vi "Move along Curve.vi"(4 "Destination Angle":dbl=nan, 5 "direction":u16(ring) items=["Clockwise", "Counter-clockwise"], 6 "Radius":dbl=5.0, 8 "error in":errorcluster, 9 "Speed":dbl=5.0, 10 "Destination":refnum<class "Vec3d.lvclass">, 11 "Gantry in":refnum<class "Gantry.lvclass">) -> (0 "error out":errorcluster, 3 "Gantry out":refnum<class "Gantry.lvclass">)   [LabVIEW 2026, in "Gantry.lvclass"]
uses:
  Gantry.lvclass
  Vec3d Class/Vec3d.lvclass
  Gantry.lvclass/Gantry.ctl
  <instrlib>/Aerotech Automation1/Tasks/Task State.ctl
  <instrlib>/Aerotech Automation1/Aerotech Automation1.lvlib
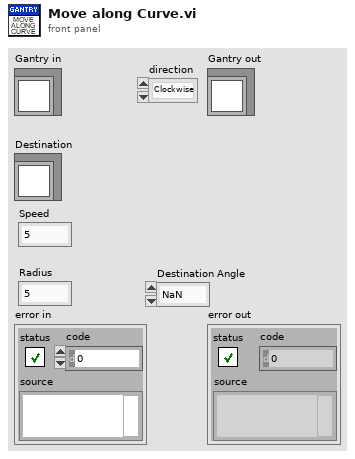
[diagram p1: front panel]
types:
  T1 = typedef "Aerotech Automation1.lvlib/Task State.ctl" = enum16{"Unavailable", "Inactive", "Idle", "ProgramReady", "ProgramRunning", "ProgramFeedhold", "ProgramPaused", "ProgramComplete", "Error", "Queue"}
  T2 = typedef "TaskStatus.ctl" = cluster{"Task Status0 (num)":i32, "Task Status0 (bits)":cluster{"CallbackHoldActive":bool, "CallbackResponding":bool, "CannedFunctionExecuting":bool, "CornerRounding":bool, "FeedHoldActive":bool, "ImmediateConcurrent":bool, "ImmediateExecuting":bool, "InterruptMotionActive":bool, "JoystickActive":bool, "JoystickLowSpeedActive":bool, "None":bool, "PendingAxesStop":bool, "ProbeCycle":bool, "ProgramAssociated":bool, "ProgramControlRestricted":bool, "ProgramReset":bool, "Retrace":bool, "ReturnMotionExecuting":bool, "SingleStepInto":bool, "SingleStepOver":bool, "SoftHomeActive":bool, "SoftwareESTOPActive":bool, "SpindleActive0":bool, "SpindleActive1":bool, "SpindleActive2":bool, "SpindleActive3":bool}, "Task Status0 (str)":string, "Task Status1 (num)":i32, "Task Status1 (bits)":cluster{"AsyncSMCMotionAbortPending":bool, "CannedFunctionPending":bool, "CutterOffsetsDisabling":bool, "CutterOffsetsEnablingNegative":bool, "CutterOffsetsEnablingPositive":bool, "CutterRadiusDisabling":bool, "CutterRadiusEnabling":bool, "FeedHeldAxesStopped":bool, "GalvoIFVDeactivationPending":bool, "IFOVBufferHold":bool, "Interrupted":bool, "MotionModeAbsOffsets":bool, "MSOChange":bool, "NoMFOFloor":bool, "None":bool, "OnGosubPending":bool, "ProgramStopPending":bool, "RetraceRequested":bool, "SpindleFeedHeld":bool}, "Task Status1 (str)":string, "Task Status2 (num)":i32, "Task Status2 (bits)":cluster{"Coord1Plane1":bool, "Coord1Plane2":bool, "Coord1Plane3":bool, "Coord2Plane1":bool, "Coord2Plane2":bool, "Coord2Plane3":bool, "CutterOffsetsActiveNeg":bool, "CutterOffsetsActivePos":bool, "CutterRadiusActiveLeft":bool, "CutterRadiusActiveRight":bool, "LimitFeedRateActive":bool, "LimitMFOActive":bool, "MirrorActive":bool, "MotionContinuousActive":bool, "MotionFiber":bool, "MotionModeCCW":bool, "MotionModeCoordinated":bool, "MotionModeCW":bool, "MotionModeRapid":bool, "MotionPVT":bool, "None":bool, "NormalcyActiveLeft":bool, "NormalcyActiveRight":bool, "NormalcyAlignment":bool, "OffsetFixtureActive":bool, "ProfileActive":bool, "RotationActive":bool, "RThetaCylindricalActive":bool, "RThetaPolarActive":bool, "ScalingActive":bool}, "Task Status2 (str)":string, "Task Mode (num)":i32, "Task Mode (bits)":cluster{"Absolute":bool, "AccelModeRate":bool, "AccelTypeLinear":bool, "AccelTypeScurve":bool, "AutoMode":bool, "BlockDelete":bool, "BlockDelete2":bool, "DecelModeRate":bool, "DecelTypeLinear":bool, "DecelTypeScurve":bool, "InverseCircular":bool, "InverseDominance":bool, "MFOActiveOnJog":bool, "MFOLock":bool, "Minutes":bool, "MotionContinuous":bool, "MSOLock":bool, "None":bool, "OptionalPause":bool, "OverMode":bool, "ProgramFeedRateMPU":bool, "ProgramFeedRateUPR":bool, "Secondary":bool, "SpindleStopOnProgramHalt":bool, "WaitAuto":bool, "WaitForInPos":bool}, "Task Mode (str)":string, "Queue Status (num)":i32, "Queue Status (bits)":cluster{"None":bool, "QueueBufferEmpty":bool, "QueueBufferFull":bool, "QueueBufferPaused":bool, "QueueBufferStarted":bool, "QueueLargeProgramExecuting":bool, "QueueModeActive":bool}, "Queue Status (str)":string, "Task State":i32}
  T3 = typedef "Aerotech Automation1.lvlib/Task Status Cluster.ctl" = cluster{"TaskState":T1, "TaskMode":i32, "AeroScriptSourceFileName":string, "CompiledAeroScriptFileName":string, "ManualFeedrateOverride":dbl, "Warning Number":i32, "Warning Message":string, "Error Number":i32, "Error Message":string}
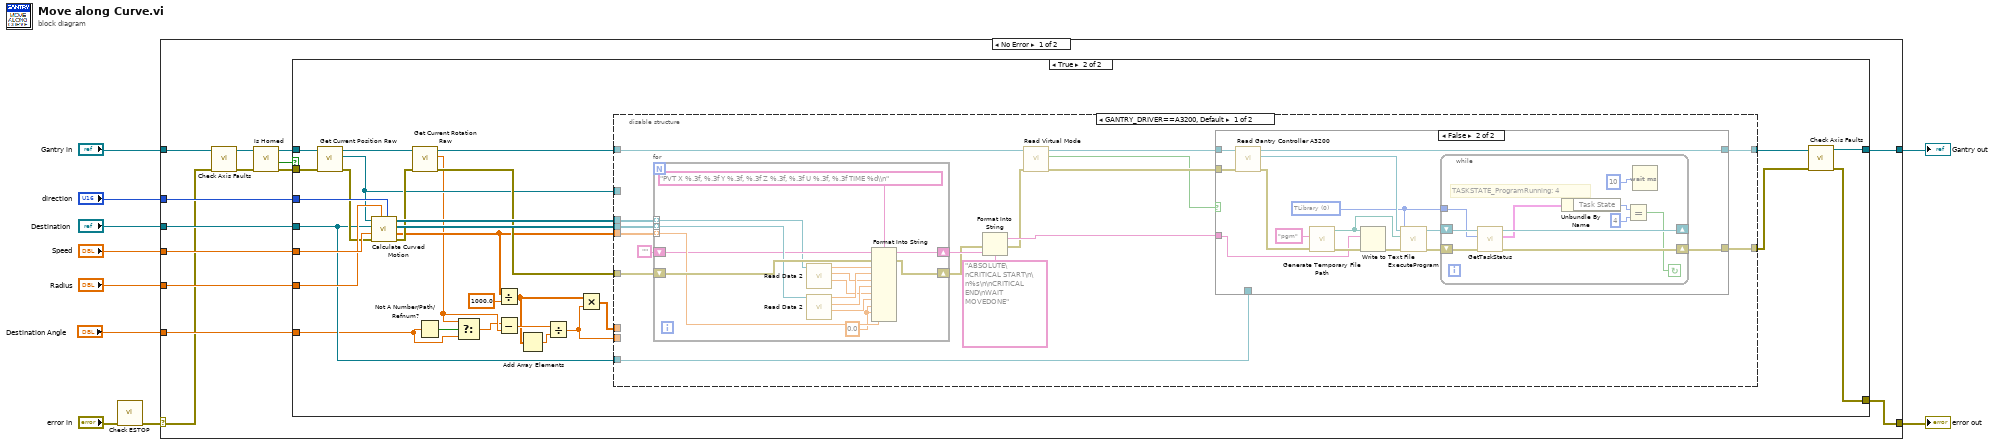
[diagram p0: block diagram]
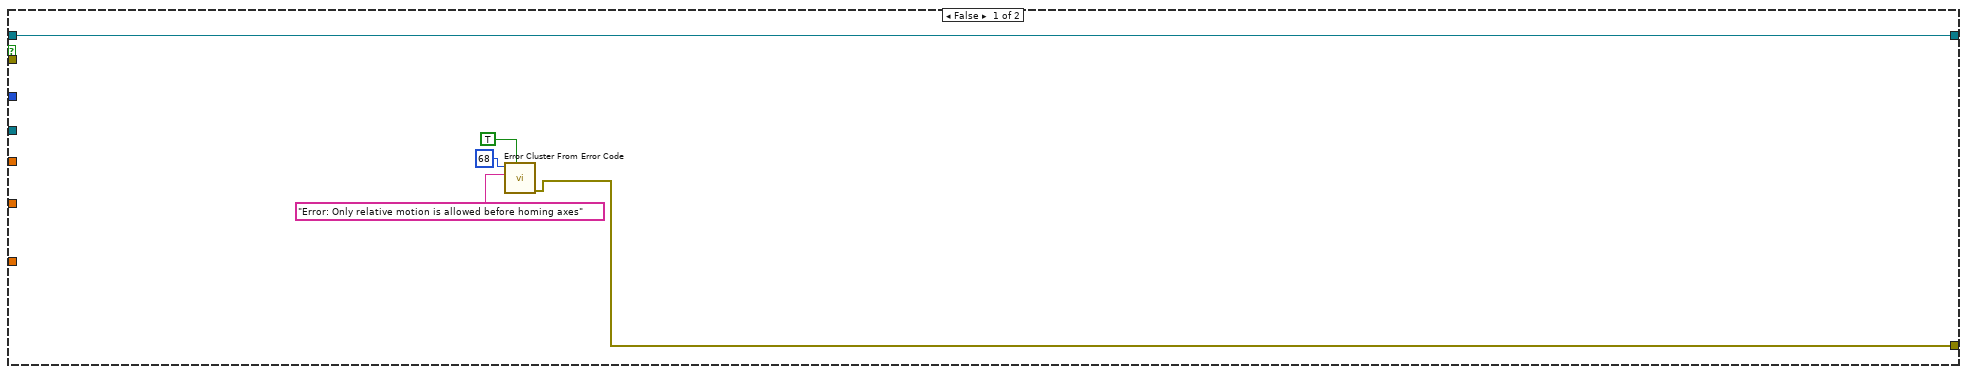
[diagram p2: hidden frame]
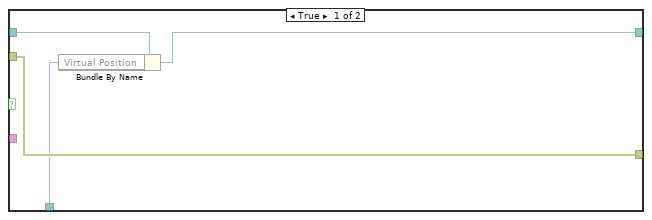
[diagram p3: hidden frame]
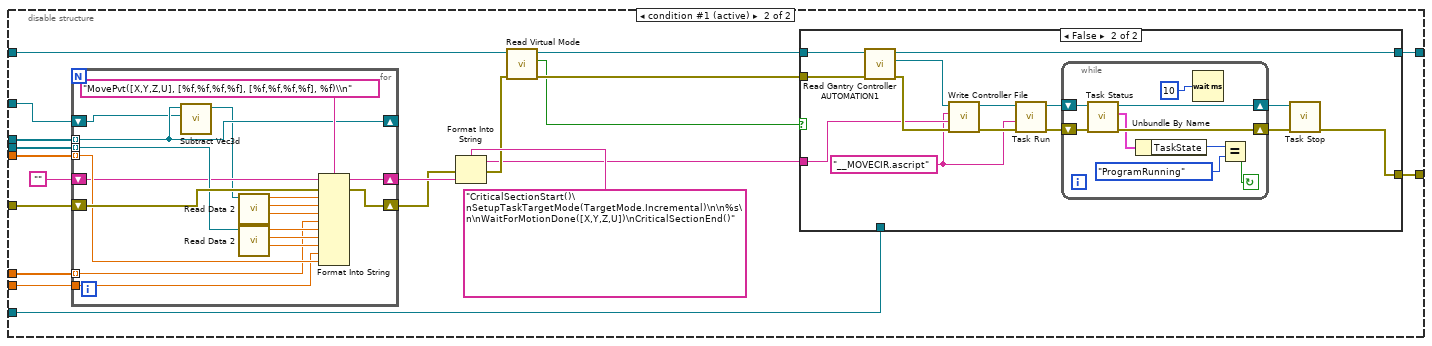
[diagram p4: hidden frame]
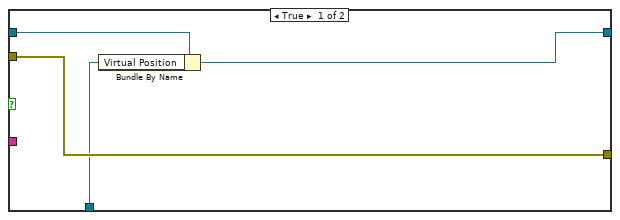
[diagram p5: hidden frame]
diagram:
  n1 = call "Check ESTOP.vi"("error in"="error in") -> ("error out"=w5:errorcluster)  [unwired: 10 in]
  n2 = case shown="No Error" w5 {
    selector: w5 -> [w14 w185]
    tunnel: [w21 w185] -> w10
    tunnel: [w22 w184] -> w9
    tunnel: "Gantry in" -> [w12 w184]
    tunnel: "Destination" -> [w24 _]
    tunnel: "Speed" -> [w23 _]
    tunnel: "direction" -> [w17 _]
    tunnel: "Radius" -> [w16 _]
    tunnel: "Destination Angle" -> [w15 _]
    frame No Error {
      n3 = call "Check Axis Faults.vi"("error in (no error)"=w14, "Gantry in"=w12) -> ("error out"=w13:errorcluster, "Gantry out"=w11:refnum<class "Gantry.lvclass">)  [unwired: 8 in]
      n4 = call "Is Homed.vi"("error in (no error)"=w13, "Gantry in"=w11) -> ("error out"=w18:errorcluster, "homed?"=w19:bool, "Gantry out"=w20:refnum<class "Gantry.lvclass">)  [unwired: 7 in]
      n5 = case shown="True" w19 {
        tunnel: w24 -> [_ w41]
        tunnel: w20 -> [w25 w43]
        tunnel: w23 -> [_ w58]
        tunnel: w18 -> [_ w42]
        tunnel: [w25 w54] -> w22
        tunnel: [w26 w52] -> w21
        tunnel: w17 -> [_ w56]
        tunnel: w16 -> [_ w57]
        tunnel: w15 -> [_ w32]
        frame False {
          n6 = call <vilib>:"Error Cluster From Error Code.vi"("show call chain? (False)"=TRUE, "error message (\"\")"="Error: Only relative motion is allowed before homing axes", "error code (0)"=68) -> ("error out"=w26:errorcluster)  [unwired: 6 in]
        }
        frame True {
          n7 = call-dynamic "Get Current Position Raw.vi"("error in"=w42, "Gantry in"=w43) -> ("error out"=w50:errorcluster, "Vec3d Class out"=w44:refnum<class "Vec3d.lvclass">, "Gantry out"=w51:refnum<class "Gantry.lvclass">)  [unwired: 7 in]
          n8 = call "Calculate Curved Motion.vi"("orientation"=w56, "Radius (mm)"=w57, "error in (no error)"=w50, "Speed (mm/s)"=w58, "Destination (mm)"=w41, "Origin (mm)"=w44) -> ("error out"=w46:errorcluster, "Times (ms)"=w36:dbl[], "Speeds (mm/s)"=w47:refnum<class "Vec3d.lvclass">[], "Coordinates (mm)"=w48:refnum<class "Vec3d.lvclass">[])  [unwired: 2 in]
          n9 = call-dynamic "Get Current Rotation Raw.vi"("error in"=w46, "Gantry in"=w51) -> ("error out"=w45:errorcluster, "Current Rotation"=w31:dbl, "Gantry out"=w49:refnum<class "Gantry.lvclass">)  [unwired: 7 in]
          n10 = Not A Number/Path/Refnum?(number/path/refnum=w32) -> (NaN/Path/Refnum?=w33:bool)
          n11 = Select(t=w31, s=w33, f=w32) -> (s? t:f=w30:dbl)
          n12 = Divide(x=w36, y=1000.0) -> (x/y=w34:dbl[])
          n13 = Subtract(x=w30, y=w31) -> (x-y=w40:dbl)
          n14 = Add Array Elements(numeric array=w34) -> (sum=w37:dbl)
          n15 = Divide(x=w40, y=w37) -> (x/y=w39:dbl)
          n16 = Multiply(x=w34, y=w39) -> (x*y=w38:dbl[])
          n17 = disable-structure shown="GANTRY_DRIVER==A3200, Default" {
            disable-tunnel: w49 -> [w66 w127]
            disable-tunnel: w48 -> [w65 w137]
            disable-tunnel: w47 -> [w64 w136]
            disable-tunnel: w36 -> [w63 w135]
            disable-tunnel: w45 -> [w62 w138]
            disable-tunnel: [w59 w131] -> w53
            disable-tunnel: [w60 w130] -> w55
            disable-tunnel: w44 -> [_ w129]
            disable-tunnel: w41 -> [w61 w122]
            disable-tunnel: w39 -> [_ w120]
            disable-tunnel: w38 -> [_ w119]
            frame condition #0 {
              n18 = for {
                shift-right: [w114] -> w71
                shift-left: w62 -> [w117]
                tunnel: w65 -> [w111] mode=indexing
                tunnel: w64 -> [w116] mode=indexing
                tunnel: w63 -> [w115] mode=indexing
                shift-right: [w112] -> w72
                shift-left: "" -> [w113]
                w104 = 0.0 ("input 4")
                n19 = call-dynamic "Read Data 2.vi"("Vec3d in"=w111) -> ("Z"=w106:dbl, "Y"=w108:dbl, "X"=w110:dbl)  [unwired: 7 in, 1 out]
                n20 = call-dynamic "Read Data 2.vi"("Vec3d in"=w116) -> ("Z"=w105:dbl, "Y"=w107:dbl, "X"=w109:dbl)  [unwired: 7 in, 1 out]
                n21 = Format Into String(format string="PVT X %.3f, %.3f Y %.3f, %.3f Z %.3f, %.3f U %.3f, %.3f TIME %d\\n", initial string=w113, error in=w117, w110, w109, w108, w107, w106, w105, w104, w104, w115) -> (resulting string=w112:string, error out=w114:errorcluster)
              }
              n22 = Format Into String(format string="ABSOLUTE\nCRITICAL START\n\n%s\n\nCRITICAL END\nWAIT MOVEDONE", error in=w71, w72) -> (resulting string=w74:string, error out=w69:errorcluster)  [unwired: 1 in]
              n23 = call-dynamic "Read Virtual Mode.vi"("error in (no error)"=w69, "Gantry in"=w66) -> ("error out"=w68:errorcluster, "Is Virtual"=w67:bool, "Gantry out"=w70:refnum<class "Gantry.lvclass">)  [unwired: 6 in, 1 out]
              n24 = case shown="False" w67 {
                tunnel: w74 -> [_ w87]
                tunnel: [w79 w81] -> w59
                tunnel: [w76 w93] -> w60
                tunnel: w70 -> [w78 w92]
                tunnel: w68 -> [w79 w91]
                tunnel: w61 -> [w77 _]
                frame True {
                  n25 = Bundle By Name(cluster=w78, "Virtual Position"=w77) -> (w76:refnum<class "Gantry.lvclass">)
                }
                frame False {
                  w80 = 0 items=["TLibrary", "T01", "T02", "T03", "T04", "T05", "T06", "T07", "T08", "T09", "T10", "T11", "T12", "T13", "T14", "T15", "T16", "T17", "T18", "T19", "T20", "T21", "T22", "T23", "T24", "T25", "T26", "T27", "T28", "T29", "T30", "T31"] ("taskId")
                  n26 = call "Read Gantry Controller A3200.vi"("error in (no error)"=w91, "Gantry in"=w92) -> ("error out"=w90:errorcluster, "A3200 controller out"=w86:refnum<k24>, "Gantry out"=w93:refnum<class "Gantry.lvclass">)  [unwired: 7 in]
                  n27 = call <vilib>:"Generate Temporary File Path.vi"("error in (no error)"=w90, "Temporary File Extension (tmp)"="pgm") -> ("error out"=w88:errorcluster, "Unique Temporary File Path"=w84:path)  [unwired: 8 in]
                  n28 = Write to Text File(file (use dialog)=w84, text=w87, error in=w88) -> (error out=w85:errorcluster)  [unwired: 1 in, 2 out]
                  n29 = call "ExecuteProgram.vi"("error in (no error)"=w85, "taskId"=w80, "program name and path"=w84, "controller in"=w86) -> ("error out"=w83:errorcluster, "controller out"=w82:refnum<k24>)  [unwired: 5 in, 1 out]
                  n30 = while {
                    shift-right: [w100] -> w81
                    shift-left: w83 -> [w102]
                    shift-right: [w101] -> _
                    shift-left: w82 -> [w103]
                    tunnel: w80 -> [w94]
                    stop <- w96 continue-if-true
                    # "TASKSTATE_ProgramRunning: 4"
                    n31 = call "GetTaskStatus.vi"("error in (no error)"=w102, "task"=w94, "controller in"=w103) -> ("error out"=w100:errorcluster, "task status"=w99:T2, "controller out"=w101:refnum<k24>)  [unwired: 6 in]
                    n32 = Unbundle By Name(w99) -> ("Task State"=w98:i32)
                    n33 = Equal?(x=w98, y=4 ("Task State")) -> (x = y?=w96:bool)
                    n34 = Wait (ms)(milliseconds to wait=u32 10) -> ()  [unwired: 1 out]
                  }
                }
              }
            }
            frame condition #1 (active) {
              n35 = for {
                shift-right: [w173] -> w128
                shift-left: w138 -> [w182]
                tunnel: w137 -> [w170] mode=indexing
                tunnel: w136 -> [w181] mode=indexing
                tunnel: w135 -> [w174] mode=indexing
                shift-right: [w171] -> w132
                shift-left: "" -> [w172]
                shift-right: [w170] -> _
                shift-left: w129 -> [w169]
                tunnel: w120 -> [w167]
                tunnel: w119 -> [w166] mode=indexing
                n36 = call "Subtract Vec3d.vi"("Vec3d in 2"=w169, "Vec3d in 1"=w170) -> ("Vec3d Class out"=w168:refnum<class "Vec3d.lvclass">)  [unwired: 8 in, 1 out]
                n37 = call-dynamic "Read Data 2.vi"("Vec3d in"=w168) -> ("Z"=w178:dbl, "Y"=w179:dbl, "X"=w180:dbl)  [unwired: 7 in, 1 out]
                n38 = call-dynamic "Read Data 2.vi"("Vec3d in"=w181) -> ("Z"=w175:dbl, "Y"=w176:dbl, "X"=w177:dbl)  [unwired: 7 in, 1 out]
                n39 = Format Into String(format string="MovePvt([X,Y,Z,U], [%f,%f,%f,%f], [%f,%f,%f,%f], %f)\\n", initial string=w172, error in=w182, w180, w179, w178, w166, w177, w176, w175, w167, w174) -> (resulting string=w171:string, error out=w173:errorcluster)
              }
              n40 = Format Into String(format string="CriticalSectionStart()\nSetupTaskTargetMode(TargetMode.Incremental)\n\n%s\n\nWaitForMotionDone([X,Y,Z,U])\nCriticalSectionEnd()", error in=w128, w132) -> (resulting string=w121:string, error out=w125:errorcluster)  [unwired: 1 in]
              n41 = call-dynamic "Read Virtual Mode.vi"("error in (no error)"=w125, "Gantry in"=w127) -> ("error out"=w124:errorcluster, "Is Virtual"=w123:bool, "Gantry out"=w126:refnum<class "Gantry.lvclass">)  [unwired: 6 in, 1 out]
              n42 = case shown="False" w123 {
                tunnel: w121 -> [_ w151]
                tunnel: [w142 w143] -> w131
                tunnel: [w139 w156] -> w130
                tunnel: w126 -> [w141 w155]
                tunnel: w124 -> [w142 w154]
                tunnel: w122 -> [w140 _]
                frame True {
                  n43 = Bundle By Name(cluster=w141, "Virtual Position"=w140) -> (w139:refnum<class "Gantry.lvclass">)
                }
                frame False {
                  w146 = "__MOVECIR.ascript" ("Controller Filename")
                  n44 = call "Read Gantry Controller AUTOMATION1.vi"("error in (no error)"=w154, "Gantry in"=w155) -> ("error out"=w152:errorcluster, "Controller AUTOMATION1"=w153:refnum<k24>, "Gantry out"=w156:refnum<class "Gantry.lvclass">)  [unwired: 7 in]
                  n45 = call <instrlib>:"Write Controller File.vi"("error in (no error)"=w152, "File Contents"=w151, "controllerFileName"=w146, "Controller Refnum in"=w153) -> ("error out"=w149:errorcluster, "Controller Refnum out"=w150:refnum<k24>)  [unwired: 6 in]
                  n46 = call <instrlib>:"Task Run.vi"("error in (no error)"=w149, "Controller Filename"=w146, "Controller Refnum"=w150) -> ("error out"=w147:errorcluster, "Controller Refnum out"=w148:refnum<k24>)  [unwired: 7 in]
                  n47 = while {
                    shift-right: [w162] -> w144
                    shift-left: w147 -> [w164]
                    shift-right: [w163] -> w145
                    shift-left: w148 -> [w165]
                    stop <- w160 continue-if-true
                    n48 = call <instrlib>:"Task Status.vi"("error in (no error)"=w164, "Controller Refnum"=w165) -> ("error out"=w162:errorcluster, "Task Status Cluster"=w161:T3, "Controller Refnum out"=w163:refnum<k24>)  [unwired: 7 in]
                    n49 = Unbundle By Name(w161) -> ("TaskState"=w159:T1)
                    n50 = Wait (ms)(milliseconds to wait=u32 10) -> ()  [unwired: 1 out]
                    n51 = Equal?(x=w159, y=Task_State."ProgramRunning" ("TaskState")) -> (x = y?=w160:bool)
                  }
                  n52 = call <instrlib>:"Task Stop.vi"("error in (no error)"=w144, "Controller Refnum"=w145) -> ("error out"=w143:errorcluster)  [unwired: 8 in, 1 out]
                }
              }
            }
          }
          n53 = call "Check Axis Faults.vi"("error in (no error)"=w53, "Gantry in"=w55) -> ("error out"=w52:errorcluster, "Gantry out"=w54:refnum<class "Gantry.lvclass">)  [unwired: 8 in]
        }
      }
    }
    frame Error {
    }
  }
  "error out" <- w10
  "Gantry out" <- w9
